vi "HW4p1_nguyejk.vi"() -> ()   [LabVIEW 2016]
panel:
  out "PE":dbl
  out "KE":dbl
  out "acceleration":dbl
  out "Velocity":dbl
  out "displacement":dbl
  in  "Time":dbl
  in  "Mass of suspended object and spring":dbl
  in  "Spring constant":dbl
  in  "Inital displacement of object":dbl
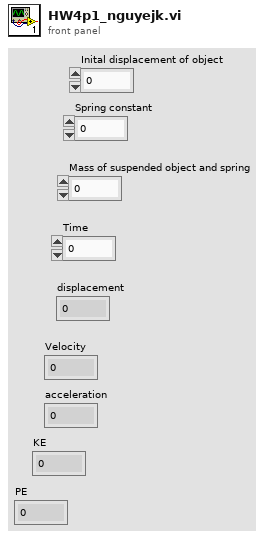
[diagram p1: front panel]
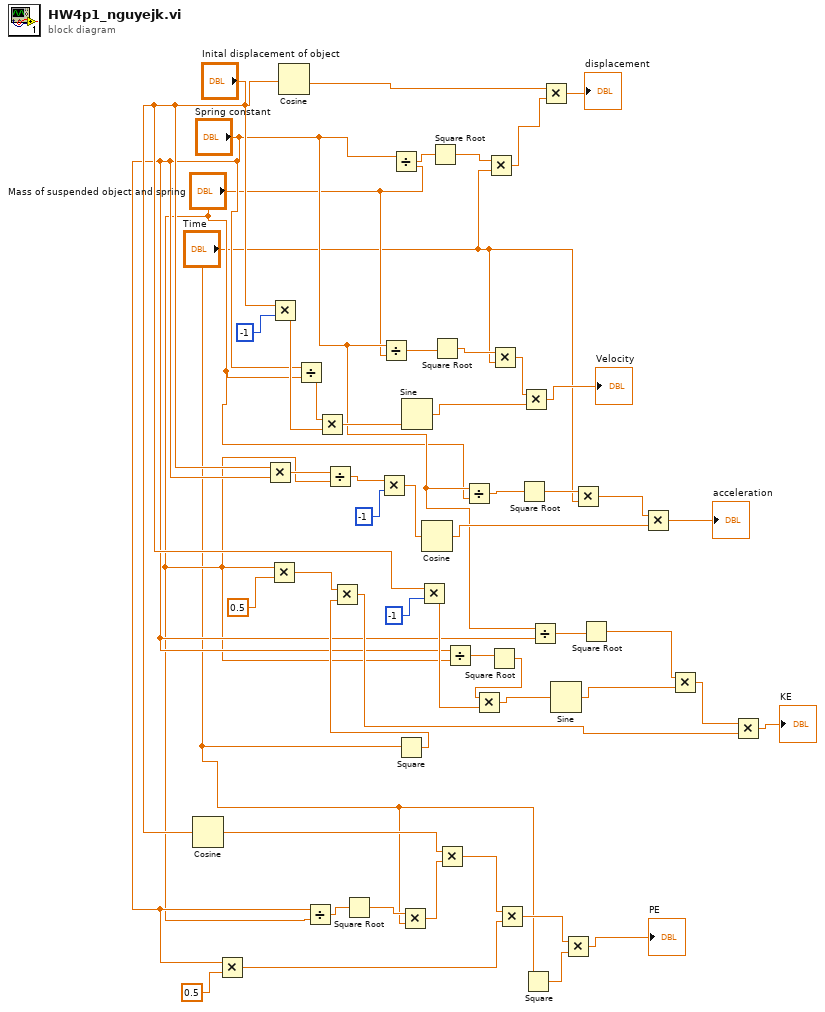
[diagram p0: block diagram]
diagram:
  n1 = Cosine(x="Inital displacement of object") -> (cos(x)=w8:dbl)
  n2 = Multiply(x="Spring constant", y=0.5) -> (x*y=w6:dbl)
  n3 = Multiply(x="Inital displacement of object", y="Spring constant") -> (x*y=w37:dbl)
  n4 = Multiply(x="Mass of suspended object and spring", y=0.5) -> (x*y=w27:dbl)
  n5 = Multiply(x="Inital displacement of object", y=-1) -> (x*y=w41:dbl)
  n6 = Cosine(x="Inital displacement of object") -> (cos(x)=w48:dbl)
  n7 = Divide(x="Spring constant", y="Mass of suspended object and spring") -> (x/y=w42:dbl)
  n8 = Divide(x="Spring constant", y="Mass of suspended object and spring") -> (x/y=w14:dbl)
  n9 = Multiply(x=w42, y=w41) -> (x*y=w43:dbl)
  n10 = Divide(x=w37, y="Mass of suspended object and spring") -> (x/y=w35:dbl)
  n11 = Square Root(x=w14) -> (sqrt(x)=w13:dbl)
  n12 = Multiply(x=w35, y=-1) -> (x*y=w32:dbl)
  n13 = Divide(x="Spring constant", y="Mass of suspended object and spring") -> (x/y=w45:dbl)
  n14 = Divide(x="Spring constant", y="Mass of suspended object and spring") -> (x/y=w51:dbl)
  n15 = Square(x="Time") -> (x^2=w19:dbl)
  n16 = Multiply(x=w27, y=w19) -> (x*y=w18:dbl)
  n17 = Multiply(x=w13, y="Time") -> (x*y=w7:dbl)
  n18 = Sine(x=w43) -> (sin(x)=w39:dbl)
  n19 = Multiply(x="Inital displacement of object", y=-1) -> (x*y=w21:dbl)
  n20 = Cosine(x=w32) -> (cos(x)=w31:dbl)
  n21 = Square Root(x=w51) -> (sqrt(x)=w50:dbl)
  n22 = Square Root(x=w45) -> (sqrt(x)=w44:dbl)
  n23 = Multiply(x=w8, y=w7) -> (x*y=w5:dbl)
  n24 = Divide(x="Spring constant", y="Mass of suspended object and spring") -> (x/y=w23:dbl)
  n25 = Divide(x="Spring constant", y="Mass of suspended object and spring") -> (x/y=w34:dbl)
  n26 = Multiply(x=w50, y="Time") -> (x*y=w49:dbl)
  n27 = Square Root(x=w23) -> (sqrt(x)=w22:dbl)
  n28 = Multiply(x=w22, y=w21) -> (x*y=w20:dbl)
  n29 = Multiply(x=w44, y="Time") -> (x*y=w40:dbl)
  n30 = Multiply(x=w5, y=w6) -> (x*y=w3:dbl)
  n31 = Square Root(x=w34) -> (sqrt(x)=w33:dbl)
  n32 = Multiply(x=w40, y=w39) -> (x*y=→"Velocity":dbl)
  n33 = Square(x="Time") -> (x^2=w4:dbl)
  n34 = Divide(x="Spring constant", y="Spring constant") -> (x/y=w25:dbl)
  n35 = Multiply(x=w48, y=w49) -> (x*y=→"displacement":dbl)
  n36 = Sine(x=w20) -> (sin(x)=w24:dbl)
  n37 = Multiply(x=w3, y=w4) -> (x*y=→"PE":dbl)
  n38 = Multiply(x=w33, y="Time") -> (x*y=w30:dbl)
  n39 = Square Root(x=w25) -> (sqrt(x)=w15:dbl)
  n40 = Multiply(x=w30, y=w31) -> (x*y=→"acceleration":dbl)
  n41 = Multiply(x=w15, y=w24) -> (x*y=w17:dbl)
  n42 = Multiply(x=w17, y=w18) -> (x*y=→"KE":dbl)
